vi "Handle ExcuseNotes.vi"(8 "error in (no error)":errorcluster, 11 "ExcuseNotes.lvclass":refnum<class "ExcuseNotesHandler.lvclass">) -> (0 "error out":errorcluster, 3 "ExcuseNotes.lvclass Out":refnum<class "ExcuseNotesHandler.lvclass">)   [LabVIEW 2015, in "Admin_Actor.lvlib"]
uses:
  Admin_Actor.lvlib
  ExcuseNotes/ExcuseNotesHandler.lvclass
  ExcuseNotes/Type Definitions/Main Ctls And VI Refs.ctl
  ListSelection.lvclass
  ExcuseNotes/ExcuseNotesHandler.lvclass/ExcuseNotesHandler.ctl
  <vilib>/Utility/error.llb/Error Cluster From Error Code.vi
  <vilib>/Utility/inputDevices.llb/mouseAcquire.vi
  <vilib>/ErrorRing/Error Ring.xnode
panel:
  in  "Commit":bool
  in  "SelectAll":bool
  in  "是否同意":bool
  in  "Name":string(combo)
  in  "Stop":bool
  in  "Table Control":string[][](table)
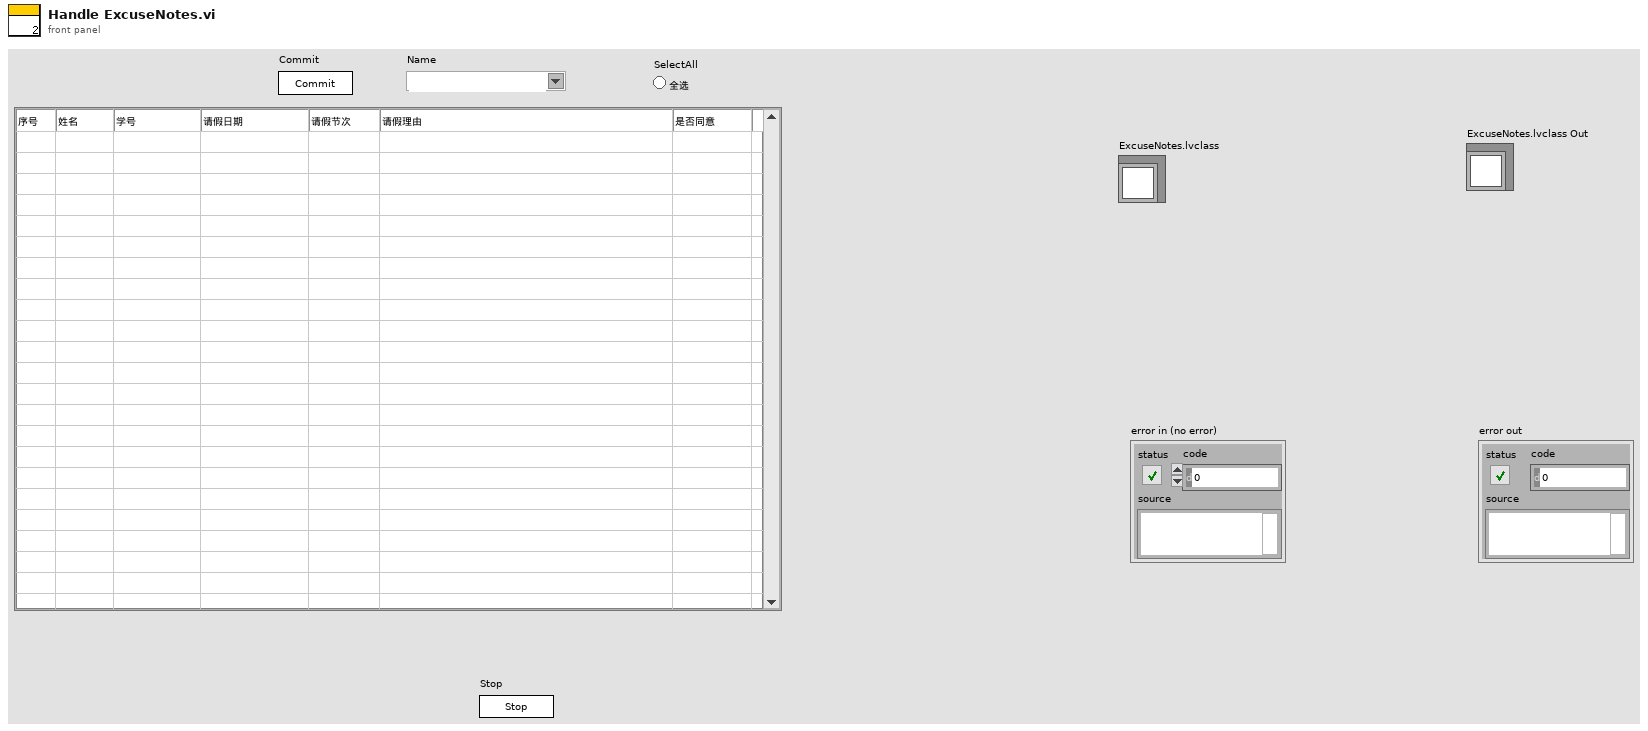
[diagram p1: front panel]
types:
  T1 = typedef "Admin_Actor.lvlib/ExcuseNotesHandler.lvclass/Main Ctls And VI Refs.ctl" = cluster{"Table Control":refnum<vi>, "Stop":refnum<vi>, "是否同意":refnum<vi>, "Name":refnum<vi>, "全选":refnum<vi>, "VI Refnum":refnum<vi>}
  T2 = enum32{"Invalid", "Standard", "Closed", "Hidden", "Minimized", "Maximized"}
  T3 = cluster{"Horizontal":i32, "Vertical":i32, "Scrolling":i32}
  T4 = typedef "LVBoundsTypeDef.ctl" = cluster{"Width":u32, "Height":u32}
  T5 = typedef "LVPositionTypeDef.ctl" = cluster{"Left":i32, "Top":i32}
  T6 = typedef "LVPoint32TypeDef.ctl" = cluster{"Horizontal":i32, "Vertical":i32}
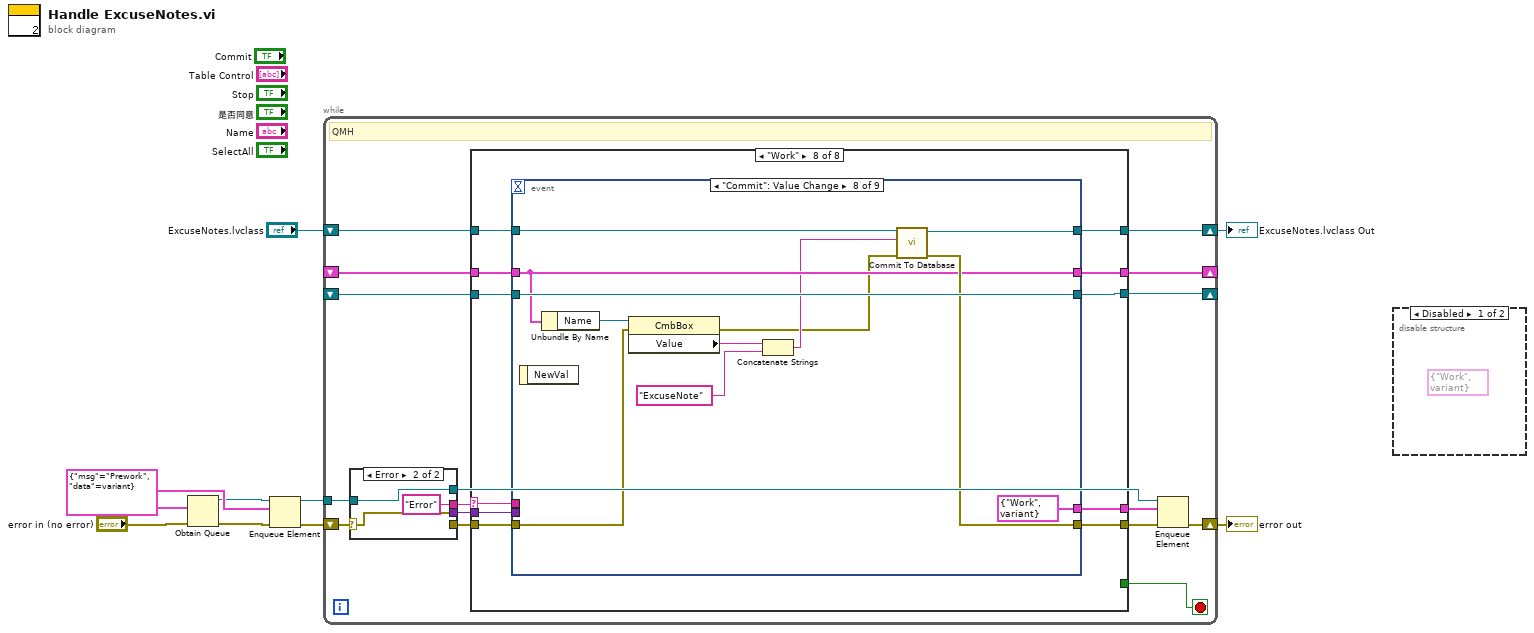
[diagram p0: block diagram]
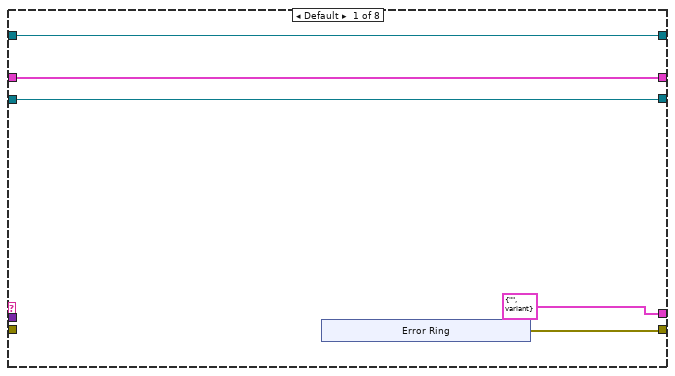
[diagram p3: hidden frame]
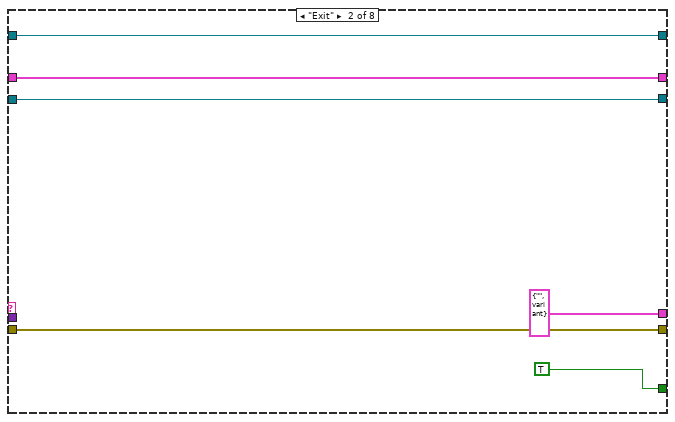
[diagram p4: hidden frame]
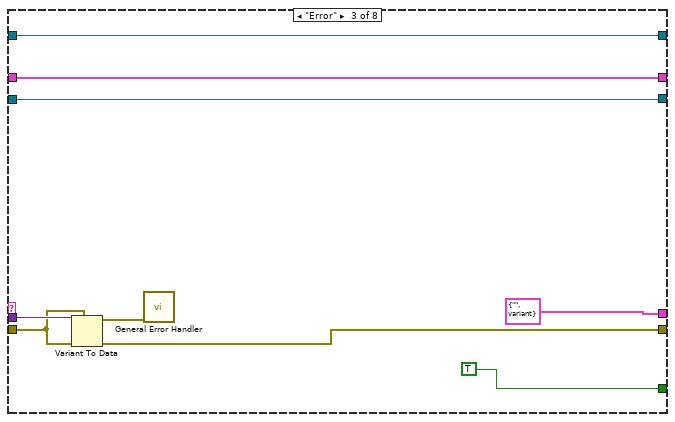
[diagram p5: hidden frame]
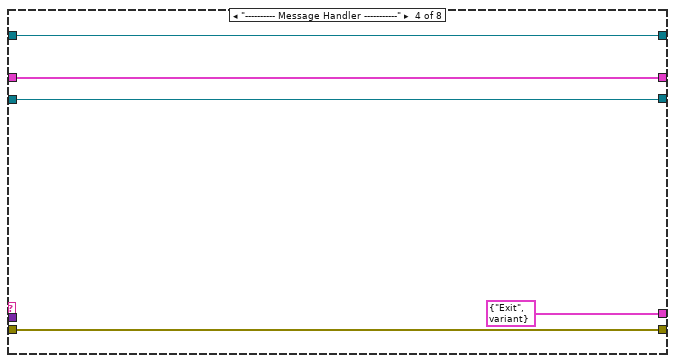
[diagram p6: hidden frame]
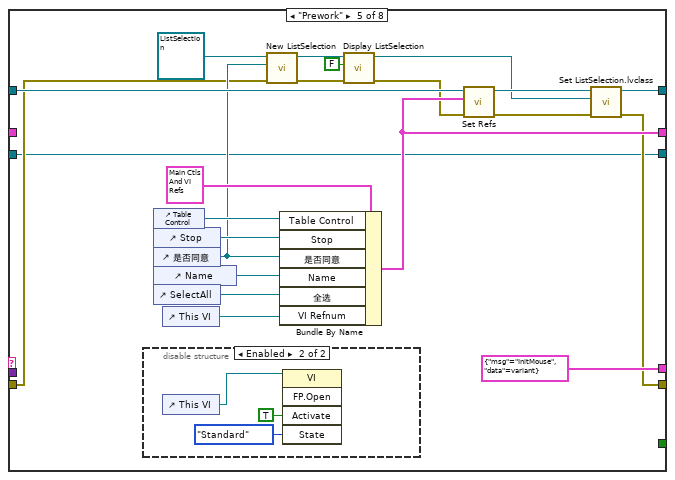
[diagram p7: hidden frame]
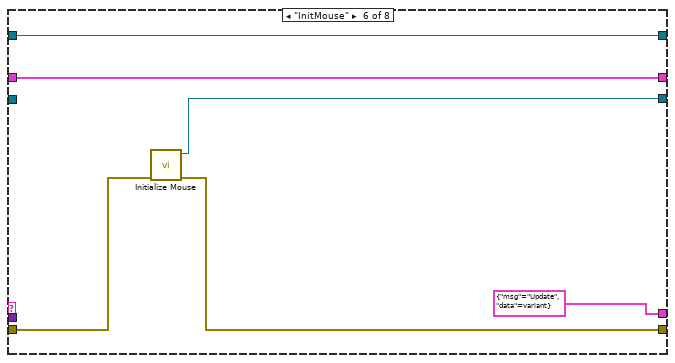
[diagram p9: hidden frame]
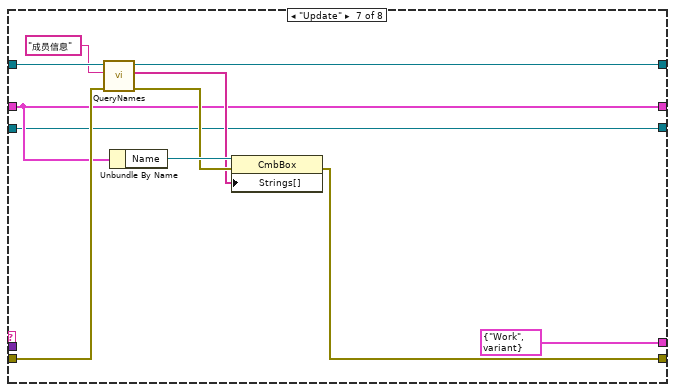
[diagram p10: hidden frame]
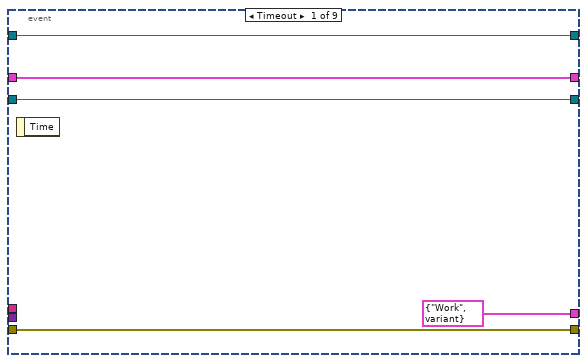
[diagram p11: hidden frame]
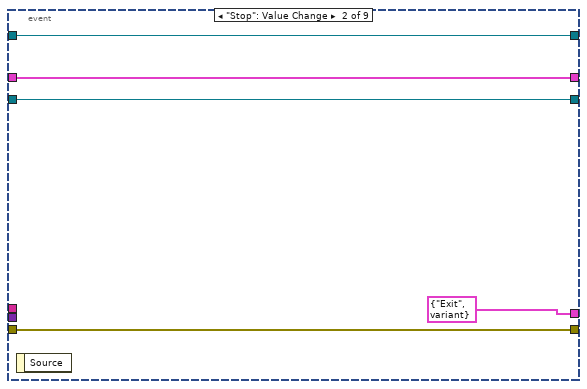
[diagram p12: hidden frame]
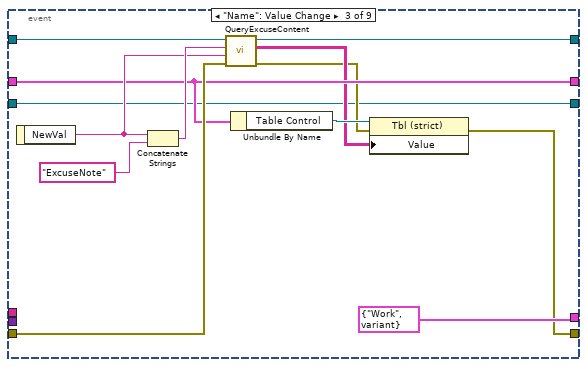
[diagram p13: hidden frame]
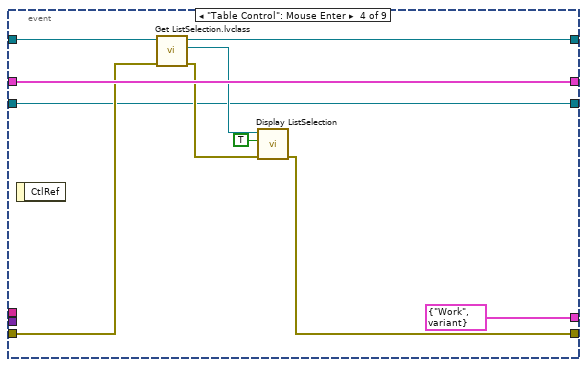
[diagram p14: hidden frame]
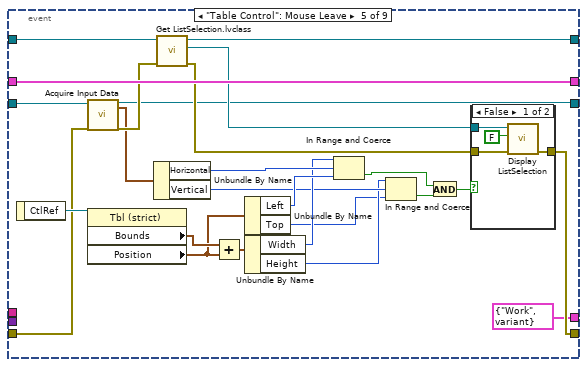
[diagram p15: hidden frame]
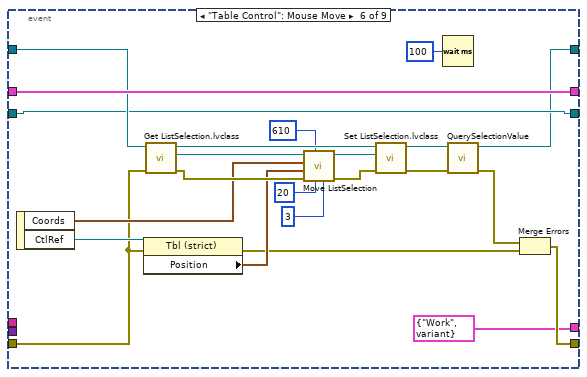
[diagram p17: hidden frame]
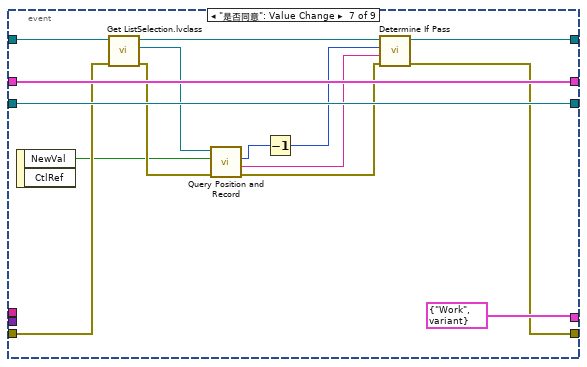
[diagram p18: hidden frame]
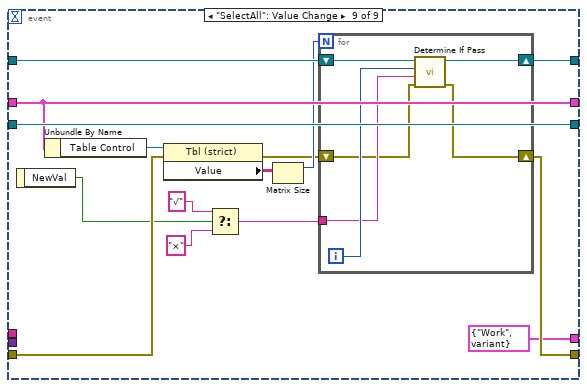
[diagram p19: hidden frame]
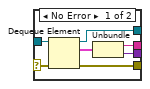
[diagram p20: hidden frame]
diagram:
  w7 = cluster{"msg":string, "data":variant} {"msg"="Prework", "data"=variant}
  n1 = Obtain Queue(element data type=w7, error in (no error)="error in (no error)") -> (queue out=w5:refnum<queue>, error out=w6:errorcluster)  [unwired: 3 in, 1 out]
  n2 = Enqueue Element(queue=w5, element=w7, error in (no error)=w6) -> (queue out=w8:refnum<queue>, error out=w9:errorcluster)  [unwired: 1 in, 1 out]
  n3 = while {
    tunnel: w8 -> [w24]
    shift-right: [w19] -> w2
    shift-left: w9 -> [w25]
    shift-right: [w14] -> w3
    shift-left: "ExcuseNotes.lvclass" -> [w15]
    shift-right: [w13] -> _
    shift-left: _ -> [w12]
    shift-right: [w11] -> _
    shift-left: _ -> [w10]
    stop <- w16 stop-if-true
    # "QMH"
    n4 = case shown="Error" w25 {
      selector: w25 -> [w248 w252]
      tunnel: w24 -> [w249 w250]
      tunnel: [w247 _] -> w23
      tunnel: [w245 "Error" ("msg")] -> w22
      tunnel: [w244 w252] -> w21
      tunnel: [w243 w250] -> w18
      frame No Error {
        n5 = Dequeue Element(queue=w249, error in (no error)=w248) -> (queue out=w243:refnum<queue>, element=w246:cluster{"msg":string, "data":variant}, error out=w247:errorcluster)  [unwired: 1 in, 1 out]
        n6 = Unbundle(w246) -> ("msg"=w245:string, "data"=w244:variant)
      }
      frame Error {
      }
    }
    n7 = case shown="\"Work\"" w22 {
      selector: w22 -> [_ _ _ _ _ _ _ w106]
      tunnel: w23 -> [_ w41 w49 w55 w62 w83 w96 w108]
      tunnel: w21 -> [_ _ w50 _ _ _ _ w107]
      tunnel: [w30 w41 w47 w55 w66 w82 w89 w105] -> w20
      tunnel: [cluster{"msg":string, "data":variant} {"msg"="", "data"=variant} cluster{"msg":string, "data":variant} {"msg"="", "data"=variant} cluster{"msg":string, "data":variant} {"msg"="", "data"=variant} cluster{"msg":string, "data":variant} {"msg"="Exit", "data"=variant} cluster{"msg":string, "data":variant} {"msg"="InitMouse", "data"=variant} cluster{"msg":string, "data":variant} {"msg"="Update", "data"=variant} cluster{"msg":string, "data":variant} {"msg"="Work", "data"=variant} w104] -> w17
      tunnel: [_ TRUE TRUE _ _ _ _ _] -> w16
      tunnel: w15 -> [w28 w38 w44 w53 w70 w86 w97 w103]
      tunnel: [w28 w38 w44 w53 w65 w86 w91 w101] -> w14
      tunnel: [w27 w37 w43 w52 w69 w85 w90 w100] -> w13
      tunnel: w12 -> [w27 w37 w43 w52 _ w85 w90 w102]
      tunnel: [w26 w36 w42 w51 w56 w81 w87 w98] -> w11
      tunnel: w10 -> [w26 w36 w42 w51 w56 _ w87 w99]
      frame Default {
        n8 = xnode ("Error Ring")() -> ("error out"=w30:errorcluster)
      }
      frame "Exit" {
      }
      frame "Error" {
        n9 = Variant To Data(error in=w49, type=w49, Variant=w50) -> (data=w48:errorcluster, error out=w47:errorcluster)
        n10 = call <vilib>:"General Error Handler.vi"("error in (no error)"=w48) -> ()  [unwired: 10 in, 5 out]
      }
      frame "---------- Message Handler -----------" {
      }
      frame "Prework" {
        n11 = disable-structure shown="Enabled" {
          frame Disabled {
          }
          frame Enabled {
            n12 = control-ref of="This VI"() -> (w80:refnum<vi>)
            n13 = invoke class="VI" method="FP.Open"(reference=w80, "Activate"=TRUE ("Activate?"), "State"=T2."Standard") -> ()  [unwired: 2 in, 5 out]
          }
        }
        n14 = control-ref of="Table Control"() -> (w75:refnum<vi>)
        n15 = control-ref of="Stop"() -> (w74:refnum<vi>)
        n16 = control-ref of="是否同意"() -> (w63:refnum<vi>)
        n17 = control-ref of="Name"() -> (w73:refnum<vi>)
        n18 = control-ref of="SelectAll"() -> (w72:refnum<vi>)
        n19 = control-ref of="This VI"() -> (w71:refnum<vi>)
        n20 = call "New ListSelection.vi"("error in (no error)"=w62, "Bool Refnum"=w63, "ListSelection in"=refnum<class "ListSelection.lvclass"> refnum ("Admin_Actor.lvlib:ListSelection.lvclass")) -> ("error out"=w60:errorcluster, "ListSelection out"=w61:refnum<class "ListSelection.lvclass">)  [unwired: 7 in]
        n21 = Bundle By Name(cluster=T1 {"Table Control"=refnum, "Stop"=refnum, "是否同意"=refnum, "Name"=refnum, "全选"=refnum, "VI Refnum"=refnum} ("Refs"), "Table Control"=w75, "Stop"=w74, "是否同意"=w63, "Name"=w73, "全选"=w72, "VI Refnum"=w71) -> (w69:T1)
        n22 = call "Display ListSelection.vi"("error in (no error)"=w60, "Visible(False)"=FALSE, "ListSelection in"=w61) -> ("error out"=w58:errorcluster, "ListSelection out"=w59:refnum<class "ListSelection.lvclass">)  [unwired: 7 in]
        n23 = call "Set Refs.vi"("error in (no error)"=w58, "Refs"=w69, "ExcuseNotes in"=w70) -> ("error out"=w67:errorcluster, "ExcuseNotes out"=w68:refnum<class "ExcuseNotesHandler.lvclass">)  [unwired: 7 in]
        n24 = call "Set ListSelection.lvclass.vi"("error in (no error)"=w67, "Admin_Actor.lvlib:ListSelection.lvclass"=w59, "ExcuseNotesHandler in"=w68) -> ("error out"=w66:errorcluster, "ExcuseNotesHandler out"=w65:refnum<class "ExcuseNotesHandler.lvclass">)  [unwired: 7 in]
      }
      frame "InitMouse" {
        n25 = call <vilib>:"Initialize Mouse.vi"("error in (no error)"=w83) -> ("error out"=w82:errorcluster, "device ID"=w81:refnum<k1>)  [unwired: 9 in]
      }
      frame "Update" {
        n26 = call "QueryNames.vi"("error in (no error)"=w96, "TableName(\"\")"="成员信息" ("TableName(\"\")"), "ExcuseNotes in"=w97) -> ("error out"=w93:errorcluster, "Names(\"\")"=w92:string[], "ExcuseNotes out"=w91:refnum<class "ExcuseNotesHandler.lvclass">)  [unwired: 6 in]
        n27 = Unbundle By Name(w90) -> ("Name"=w94:refnum<vi>)
        n28 = property class="CmbBox"(reference=w94, error in=w93, "Strings[]"=w92) -> (error out=w89:errorcluster)  [unwired: 1 out]
      }
      frame "Work" {
        n29 = event shown="[7] \"Commit\": Value Change" {
          selector: _ -> [_ _ _ _ _ _ _ _ _]
          dyn-events: _ -> [_ _ _ _ _ _ _ _ _]
          timeout: _ -> [_ _ _ _ _ _ _ _ _]
          tunnel: w108 -> [w113 w118 w129 w139 w156 w185 w203 w214 w232]
          tunnel: w107 -> [_ _ _ _ _ _ _ _ _]
          tunnel: w106 -> [_ _ _ _ _ _ _ _ _]
          tunnel: [w113 w118 w120 w135 w162 w180 w206 w218 w223] -> w105
          tunnel: [cluster{"msg":string, "data":variant} {"msg"="Work", "data"=variant} cluster{"msg":string, "data":variant} {"msg"="Exit", "data"=variant} cluster{"msg":string, "data":variant} {"msg"="Work", "data"=variant} cluster{"msg":string, "data":variant} {"msg"="Work", "data"=variant} cluster{"msg":string, "data":variant} {"msg"="Work", "data"=variant} cluster{"msg":string, "data":variant} {"msg"="Work", "data"=variant} cluster{"msg":string, "data":variant} {"msg"="Work", "data"=variant} cluster{"msg":string, "data":variant} {"msg"="Work", "data"=variant} cluster{"msg":string, "data":variant} {"msg"="Work", "data"=variant}] -> w104
          tunnel: w103 -> [w111 w116 w130 w140 w165 w193 w204 w220 w235]
          tunnel: w102 -> [w110 w115 w124 w141 w166 w194 w209 w216 w234]
          tunnel: [w111 w116 w125 w133 w160 w173 w205 w219 w224] -> w101
          tunnel: [w110 w115 w124 w141 w166 w194 w209 w216 w234] -> w100
          tunnel: w99 -> [w109 w114 w119 w132 w157 w177 w207 w221 w236]
          tunnel: [w109 w114 w119 w132 w154 w177 w207 w221 w236] -> w98
          event Timeout {
            n30 = event-data() -> ()  [unwired: 1 in, 1 out]
          }
          event "Stop": Value Change {
            n31 = event-data() -> ()  [unwired: 1 in, 1 out]
          }
          event "Name": Value Change {
            n32 = event-data() -> ("NewVal"=w127:string)  [unwired: 1 in]
            n33 = Concatenate Strings(w127, "ExcuseNote" ("string")) -> (w128:string)
            n34 = call "QueryExcuseContent.vi"("error in (no error)"=w129, "Name"=w127, "TableName"=w128, "ExcuseNotes in"=w130) -> ("error out"=w121:errorcluster, "ExcuseNote(\"\")"=w122:string[][], "ExcuseNotes out"=w125:refnum<class "ExcuseNotesHandler.lvclass">)  [unwired: 5 in]
            n35 = Unbundle By Name(w124) -> ("Table Control"=w123:refnum<vi>)
            n36 = property class="Tbl (strict)"(reference=w123, error in=w121, "Value"=w122) -> (error out=w120:errorcluster)  [unwired: 1 out]
          }
          event "Table Control": Mouse Enter {
            n37 = event-data() -> ()  [unwired: 1 in, 1 out]
            n38 = call "Get ListSelection.lvclass.vi"("error in (no error)"=w139, "ExcuseNotesHandler in"=w140) -> ("error out"=w137:errorcluster, "Admin_Actor.lvlib:ListSelection.lvclass"=w138:refnum<class "ListSelection.lvclass">, "ExcuseNotesHandler out"=w133:refnum<class "ExcuseNotesHandler.lvclass">)  [unwired: 7 in]
            n39 = call "Display ListSelection.vi"("error in (no error)"=w137, "Visible(False)"=TRUE, "ListSelection in"=w138) -> ("error out"=w135:errorcluster)  [unwired: 7 in, 1 out]
          }
          event "Table Control": Mouse Leave {
            n40 = event-data() -> ("CtlRef"=w159:refnum<vi>)  [unwired: 1 in]
            n41 = call-poly <vilib>:"Acquire Input Data.vi"("device ID"=w157, "error in (no error)"=w156) -> ("device ID"=w154:refnum<k1>, "axis info"=w153:T3, "error out"=w155:errorcluster)  [unwired: 14 in, 1 out]
            n42 = property class="Tbl (strict)"(reference=w159) -> ("Bounds"=w158:T4, "Position"=w152:T5)  [unwired: 1 in, 2 out]
            n43 = Unbundle By Name(w153) -> ("Horizontal"=w150:i32, "Vertical"=w147:i32)
            n44 = call "Get ListSelection.lvclass.vi"("error in (no error)"=w155, "ExcuseNotesHandler in"=w165) -> ("error out"=w163:errorcluster, "Admin_Actor.lvlib:ListSelection.lvclass"=w164:refnum<class "ListSelection.lvclass">, "ExcuseNotesHandler out"=w160:refnum<class "ExcuseNotesHandler.lvclass">)  [unwired: 7 in]
            n45 = Add(x=w158, y=w152) -> (x+y=w151:T4)
            n46 = Unbundle By Name(w152) -> ("Left"=w149:i32, "Top"=w145:i32)
            n47 = Unbundle By Name(w151) -> ("Width"=w148:u32, "Height"=w146:u32)
            n48 = In Range and Coerce(upper limit=w148, x=w150, lower limit=w149) -> (In Range?=w144:bool)  [unwired: 1 out]
            n49 = In Range and Coerce(upper limit=w146, x=w147, lower limit=w145) -> (In Range?=w143:bool)  [unwired: 1 out]
            n50 = And(x=w144, y=w143) -> (x .and. y?=w142:bool)
            n51 = case shown="False" w142 {
              tunnel: w164 -> [w170 _]
              tunnel: w163 -> [w169 w171]
              tunnel: [w167 w171] -> w162
              frame False {
                n52 = call "Display ListSelection.vi"("error in (no error)"=w169, "Visible(False)"=FALSE, "ListSelection in"=w170) -> ("error out"=w167:errorcluster)  [unwired: 7 in, 1 out]
              }
              frame True {
              }
            }
          }
          event "Table Control": Mouse Move {
            n53 = event-data() -> ("Coords"=w187:T6, "CtlRef"=w186:refnum<vi>)  [unwired: 1 in]
            n54 = property class="Tbl (strict)"(reference=w186, error in=w185) -> (error out=w181:errorcluster, "Position"=w184:T5)  [unwired: 1 out]
            n55 = call "Get ListSelection.lvclass.vi"("error in (no error)"=w185, "ExcuseNotesHandler in"=w193) -> ("error out"=w189:errorcluster, "Admin_Actor.lvlib:ListSelection.lvclass"=w192:refnum<class "ListSelection.lvclass">, "ExcuseNotesHandler out"=w191:refnum<class "ExcuseNotesHandler.lvclass">)  [unwired: 7 in]
            n56 = call "Move ListSelection.vi"("Bias"=3, "Size"=20, "Herizon"=610 ("Size"), "error in (no error)"=w189, "List_Rec"=w184, "Mou_Pos"=w187, "ListSelection in"=w192) -> ("error out"=w188:errorcluster, "ListSelection out"=w190:refnum<class "ListSelection.lvclass">)  [unwired: 3 in]
            n57 = call "Set ListSelection.lvclass.vi"("error in (no error)"=w188, "Admin_Actor.lvlib:ListSelection.lvclass"=w190, "ExcuseNotesHandler in"=w191) -> ("error out"=w175:errorcluster, "ExcuseNotesHandler out"=w176:refnum<class "ExcuseNotesHandler.lvclass">)  [unwired: 7 in]
            n58 = Wait (ms)(milliseconds to wait=u32 100) -> ()  [unwired: 1 out]
            n59 = call "QuerySelectionValue.vi"("error in (no error)"=w175, "ExcuseNotesHandler in"=w176) -> ("error out"=w174:errorcluster, "ExcuseNotesHandler out"=w173:refnum<class "ExcuseNotesHandler.lvclass">)  [unwired: 8 in]
            n60 = Merge Errors(w174, w181) -> (w180:errorcluster)
          }
          event "是否同意": Value Change {
            n61 = event-data() -> ("NewVal"=w200:bool)  [unwired: 1 in, 1 out]
            n62 = call "Get ListSelection.lvclass.vi"("error in (no error)"=w203, "ExcuseNotesHandler in"=w204) -> ("error out"=w201:errorcluster, "Admin_Actor.lvlib:ListSelection.lvclass"=w202:refnum<class "ListSelection.lvclass">, "ExcuseNotesHandler out"=w199:refnum<class "ExcuseNotesHandler.lvclass">)  [unwired: 7 in]
            n63 = call "Query Position and Record.vi"("error in (no error)"=w201, "SelectKey(True)"=w200, "ListSelection in"=w202) -> ("error out"=w197:errorcluster, "SignedResult(\"\")"=w198:string, "InxOfColumns"=w196:i32)  [unwired: 5 in, 1 out]
            n64 = Decrement(x=w196) -> (x-1=w195:i32)
            n65 = call "Determine If Pass.vi"("error in (no error)"=w197, "DetermineResult(\"\")"=w198, "SelectRow(0)"=w195, "ExcuseNotesHandler in"=w199) -> ("error out"=w206:errorcluster, "ExcuseNotesHandler out"=w205:refnum<class "ExcuseNotesHandler.lvclass">)  [unwired: 6 in]
          }
          event "Commit": Value Change {
            n66 = event-data() -> ()  [unwired: 1 in, 1 out]
            n67 = Unbundle By Name(w216) -> ("Name"=w215:refnum<vi>)
            n68 = property class="CmbBox"(reference=w215, error in=w214) -> (error out=w210:errorcluster, "Value"=w213:string)  [unwired: 1 out]
            n69 = Concatenate Strings(w213, "ExcuseNote" ("string")) -> (w211:string)
            n70 = call "Commit To Database.vi"("error in (no error)"=w210, "TableName(\"\")"=w211, "ExcuseNotesHandler in"=w220) -> ("error out"=w218:errorcluster, "ExcuseNotesHandler out"=w219:refnum<class "ExcuseNotesHandler.lvclass">)  [unwired: 7 in]
          }
          event "SelectAll": Value Change {
            n71 = event-data() -> ("NewVal"=w229:bool)  [unwired: 1 in]
            n72 = Unbundle By Name(w234) -> ("Table Control"=w233:refnum<vi>)
            n73 = property class="Tbl (strict)"(reference=w233, error in=w232) -> (error out=w225:errorcluster, "Value"=w231:string[][])  [unwired: 1 out]
            n74 = Select(t="√", s=w229, f="×") -> (s? t:f=w226:string)
            n75 = Matrix Size(0:w231) -> (1:w230:i32)  [unwired: 1 out]
            n76 = for {
              N: w230 -> [_]
              tunnel: w226 -> [w240]
              shift-right: [w238] -> w224
              shift-left: w235 -> [w242]
              shift-right: [w237] -> w223
              shift-left: w225 -> [w239]
              i -> [w241]
              n77 = call "Determine If Pass.vi"("error in (no error)"=w239, "DetermineResult(\"\")"=w240, "SelectRow(0)"=w241, "ExcuseNotesHandler in"=w242) -> ("error out"=w237:errorcluster, "ExcuseNotesHandler out"=w238:refnum<class "ExcuseNotesHandler.lvclass">)  [unwired: 6 in]
            }
          }
        }
      }
    }
    n78 = Enqueue Element(queue=w18, element=w17, error in (no error)=w20) -> (error out=w19:errorcluster)  [unwired: 1 in, 2 out]
  }
  "ExcuseNotes.lvclass Out" <- w3
  "error out" <- w2
  n79 = disable-structure shown="Disabled" {
    frame Disabled {
      (unwired) cluster{"msg":string, "data":variant} {"msg"="Work", "data"=variant}
    }
    frame Enabled {
    }
  }
